vi "UART.vi"() -> ()   [LabVIEW 2024]
uses:
  <vilib>/Instr/_visa.llb/VISA Configure Serial Port (Instr).vi
panel:
  out "Boolean 2":bool
  out "Mots de passe":string
  in  "OK Button 10":bool
  in  "OK Button 9":bool
  in  "OK Button 8":bool
  in  "OK Button 7":bool
  in  "OK Button 6":bool
  in  "OK Button 4":bool
  in  "OK Button 5":bool
  in  "OK Button 3":bool
  in  "OK Button 2":bool
  out "UART":string
  in  "Data send":string
  in  "Cancel Button":bool
  in  "OK Button":bool
  in  "stop":bool
  in  "VISA resource name":refnum<visa-resource-name>
  in  "Boolean":bool
  out "Waveform Chart":dbl(graph)
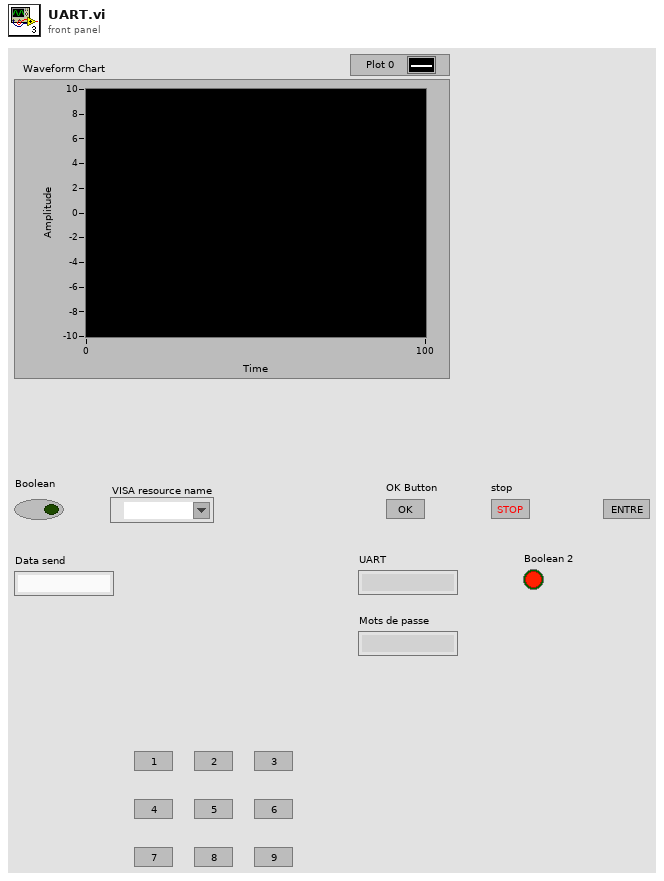
[diagram p1: front panel]
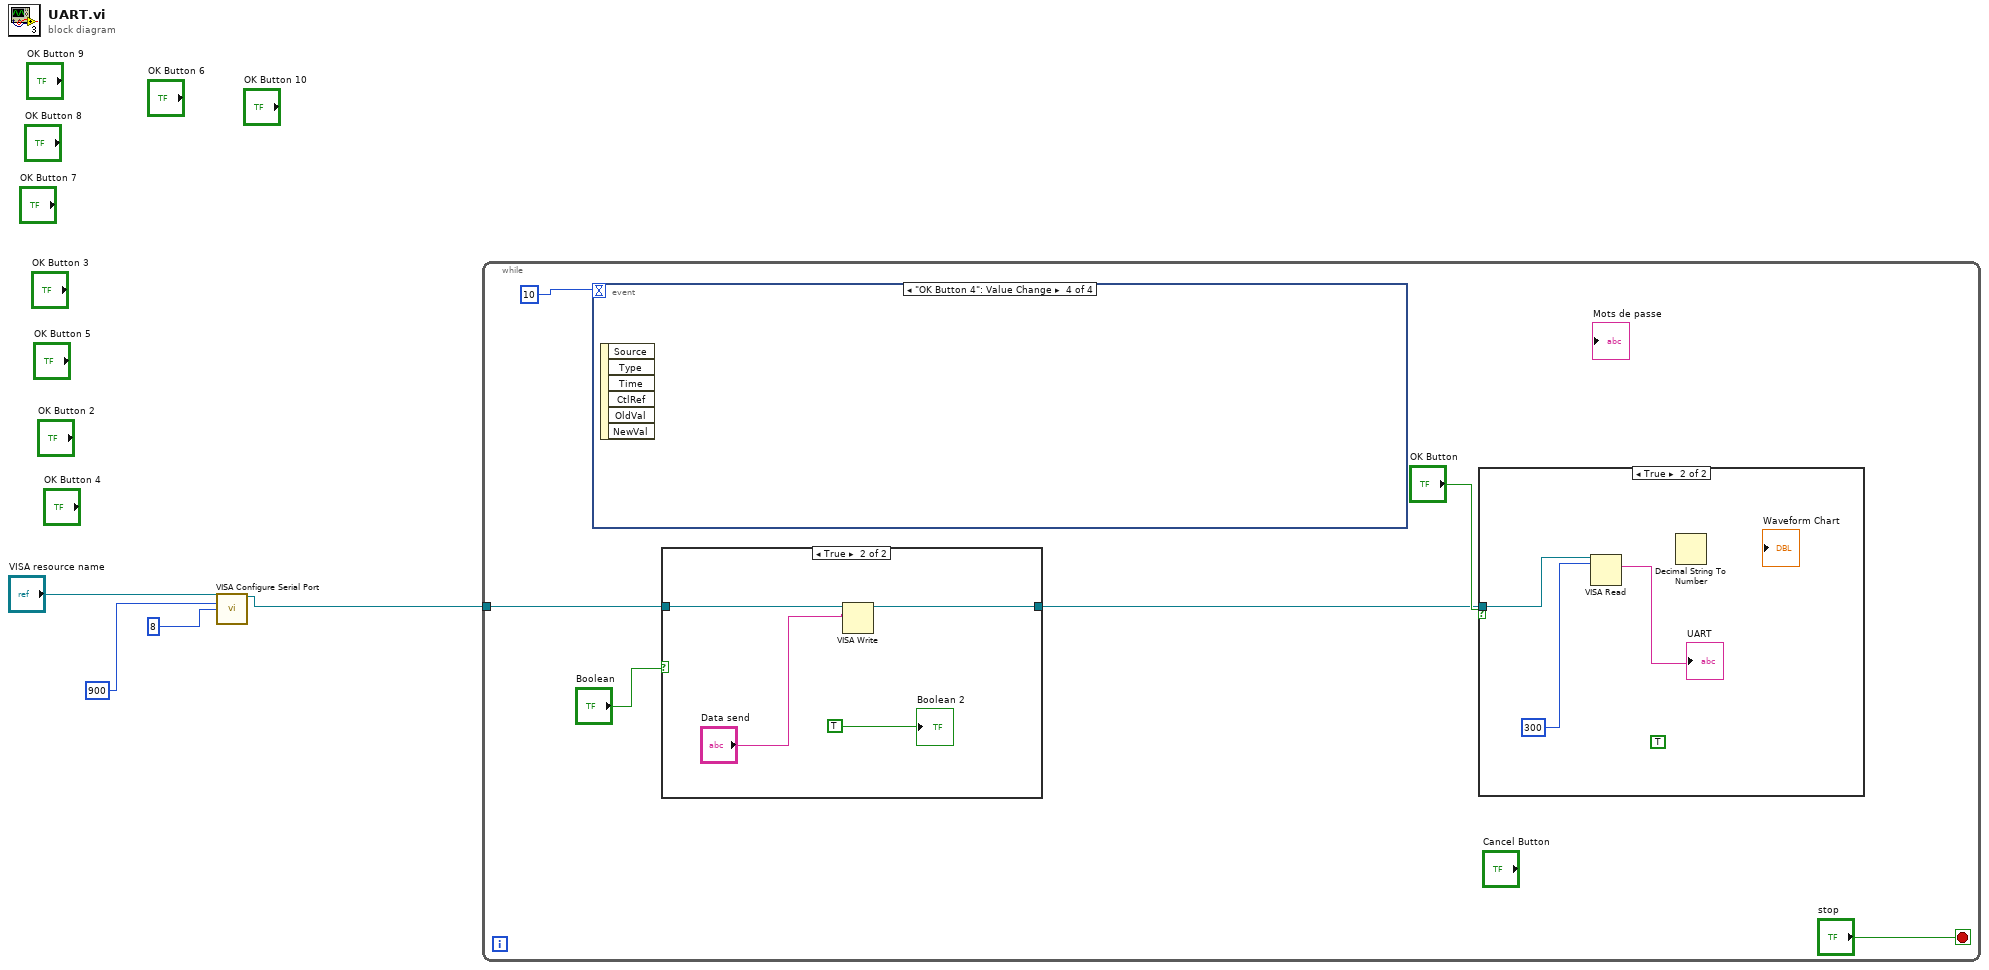
[diagram p0: block diagram]
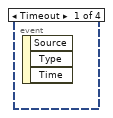
[diagram p2: hidden frame]
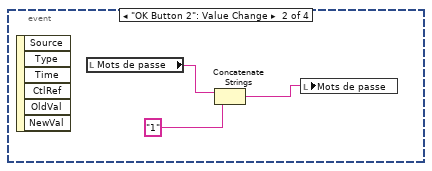
[diagram p3: hidden frame]
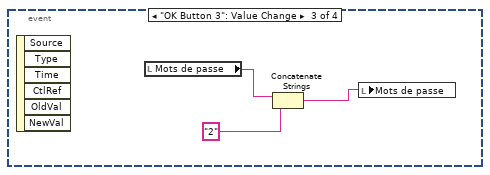
[diagram p4: hidden frame]
diagram:
  n1 = call-poly "VISA Configure Serial Port"("VISA resource name"="VISA resource name", "baud rate (9600)"=900, "data bits (8)"=8) -> ("VISA resource name out"=w1:refnum<visa-resource-name>)  [unwired: 11 in, 1 out]
  n2 = while {
    tunnel: w1 -> [w7]
    stop <- "stop" stop-if-true
    n3 = event shown="[3] \"OK Button 4\": Value Change" {
      selector: _ -> [_ _ _ _]
      dyn-events: _ -> [_ _ _ _]
      timeout: 10 -> [_ _ _ _]
      event Timeout {
        n4 = event-data() -> ()  [unwired: 1 in, 3 out]
      }
      event "OK Button 2": Value Change {
        n5 = event-data() -> ()  [unwired: 1 in, 6 out]
        n6 = local read "Mots de passe"() -> (w11:string)
        n7 = Concatenate Strings(w11, "1") -> (w13:string)
        n8 = local write "Mots de passe"(w13) -> ()
      }
      event "OK Button 3": Value Change {
        n9 = event-data() -> ()  [unwired: 1 in, 6 out]
        n10 = local read "Mots de passe"() -> (w14:string)
        n11 = Concatenate Strings(w14, "2") -> (w16:string)
        n12 = local write "Mots de passe"(w16) -> ()
      }
      event "OK Button 4": Value Change {
        n13 = event-data() -> ()  [unwired: 1 in, 6 out]
      }
    }
    n14 = case shown="True" "Boolean" {
      tunnel: w7 -> [_ w23]
      tunnel: [_ w22] -> w6
      frame False {
      }
      frame True {
        n15 = VISA Write(VISA resource name=w23, write buffer="Data send") -> (VISA resource name out=w22:refnum<visa-resource-name>)  [unwired: 1 in, 2 out]
        "Boolean 2" <- TRUE
      }
    }
    n16 = case shown="True" "OK Button" {
      tunnel: w6 -> [_ w20]
      frame False {
      }
      frame True {
        w17 = TRUE
        n17 = VISA Read(VISA resource name=w20, byte count=300) -> (read buffer=→"UART":string)  [unwired: 1 in, 3 out]
        n18 = Decimal String To Number() -> ()  [unwired: 3 in, 2 out]
      }
    }
  }
